vi "Read waveform file.vi"(7 "File IO parameters":T1={"Output Folder"=path "C:/Users/Abigail/Documents/Imperial Optical software/Optical Software Code Simplified/Output", "Error file"=path "Error Log.txt", "Config file"=path "Config.ini", "File prefix"="", "Waveform read"={"t0"=timestamp(0 s since 1904-01-01), "dt"=1.0, "Y"=[]}}, 8 "error in":errorcluster, 11 "Dataset name":string="DAQ (raw data)") -> (0 "error out":errorcluster, 2 "all rows":dbl[][](array[numeric]), 3 "Waveform":waveform(dbl))   [LabVIEW 2017, in "File IO.lvlib"]
uses:
  File IO.lvlib
  Controls/Params.ctl
  <vilib>/Utility/file.llb/Read Delimited Spreadsheet (DBL).vi
  <vilib>/Utility/file.llb/Read Delimited Spreadsheet (string).vi
panel:
  out "date last modified":timestamp
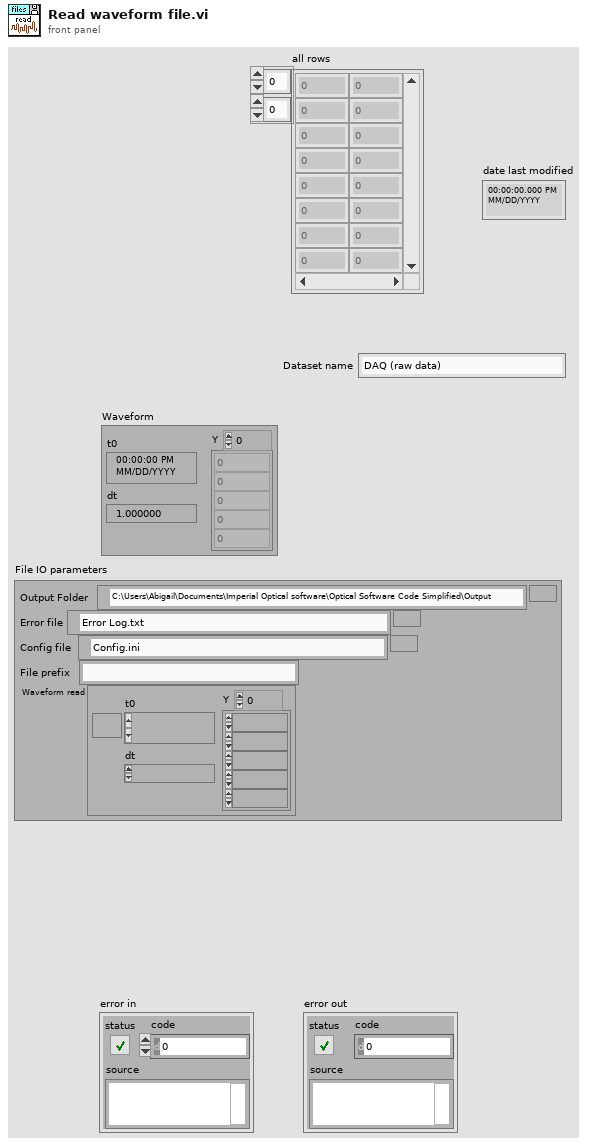
[diagram p1: front panel]
types:
  T1 = typedef "File IO.lvlib/Params.ctl" = cluster{"Output Folder":path, "Error file":path, "Config file":path, "File prefix":string, "Waveform read":waveform(dbl)}
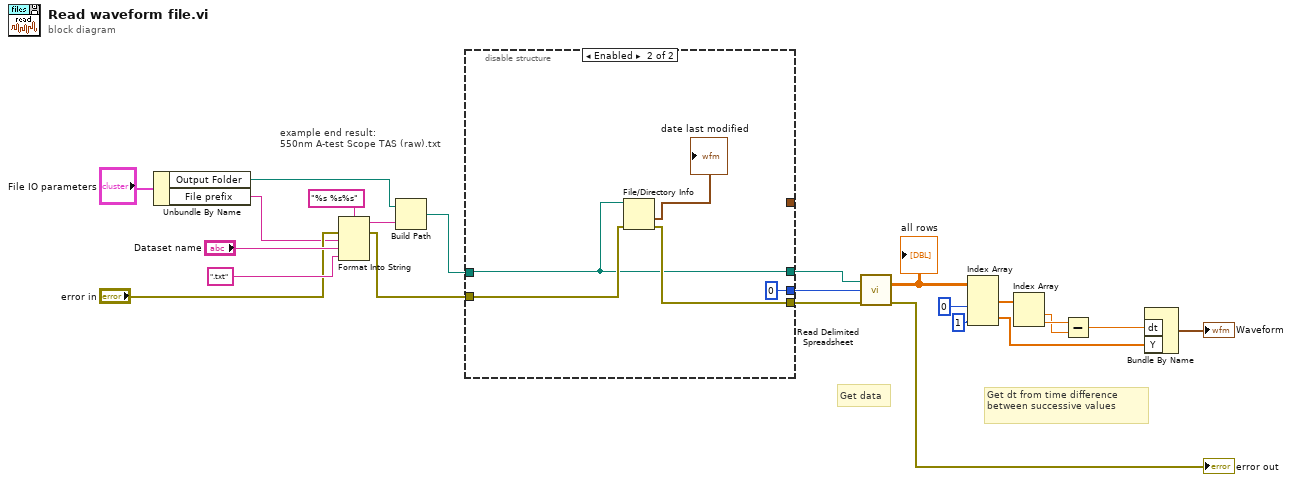
[diagram p0: block diagram]
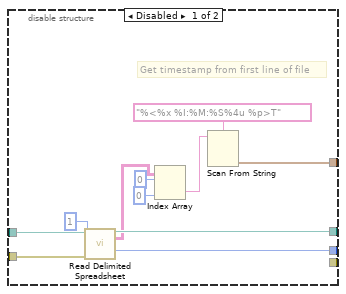
[diagram p2: hidden frame]
diagram:
  # "Get data"
  # "Get dt from time difference between successive values"
  # "example end result:\n550nm A-test Scope TAS (raw).txt"
  n1 = Unbundle By Name("File IO parameters") -> ("Output Folder"=w23:path, "File prefix"=w2:string)
  n2 = Format Into String(format string="%s %s%s", error in="error in", w2, "Dataset name", ".txt" ("Dataset name 2")) -> (resulting string=w19:string, error out=w16:errorcluster)  [unwired: 1 in]
  n3 = Build Path(base path=w23, name or relative path=w19) -> (appended path=w1:path)
  n4 = disable-structure shown="Enabled" {
    disable-tunnel: w1 -> [w34 w36]
    disable-tunnel: w16 -> [w33 w38]
    disable-tunnel: [w32 0 ("mark after read (chars.)")] -> w15
    disable-tunnel: [w31 w36] -> w14
    disable-tunnel: [w24 _] -> _
    disable-tunnel: [_ w37] -> w4
    frame Disabled {
      # "Get timestamp from first line of file"
      n5 = call-poly <vilib>:"Read Delimited Spreadsheet.vi"("file path (dialog if empty)"=w34, "number of rows (all:-1)"=1, "error in (no error)"=w33) -> ("new file path (Not A Path if cancelled)"=w31:path, "all rows"=w29:string[][], "mark after read (chars.)"=w32:i32)  [unwired: 7 in, 3 out]
      n6 = Index Array(array=w29, index (row)=0 ("disabled index (row)"), index (col)=0 ("disabled index (col)")) -> (element=w26:string)
      n7 = Scan From String(format string="%<%x %I:%M:%S%4u %p>T" ("time format string (%c)"), input string=w26) -> (output 1=w24:timestamp)  [unwired: 3 in, 3 out]
    }
    frame Enabled {
      n8 = File/Directory Info(path=w36, error in=w38) -> (last mod=→"date last modified":timestamp, error out=w37:errorcluster)  [unwired: 5 out]
    }
  }
  n9 = call-poly <vilib>:"Read Delimited Spreadsheet.vi"("file path (dialog if empty)"=w14, "start of read offset (chars.:0)"=w15, "error in (no error)"=w4) -> ("all rows"=w12:dbl[][], "error out"=→"error out":errorcluster)  [unwired: 7 in, 4 out]
  "all rows" <- w12
  n10 = Index Array(array=w12, index (col) #1=0 ("disabled index (col)"), index (col) #2=1 ("index (col)")) -> (element #1=w10:dbl[], element #2=w5:dbl[])  [unwired: 2 in]
  n11 = Index Array(array=w10) -> (element #1=w8:dbl, element #2=w9:dbl)  [unwired: 2 in]
  n12 = Subtract(x=w9, y=w8) -> (x-y=w7:dbl)
  n13 = Bundle By Name("dt"=w7, "Y"=w5) -> (→"Waveform":waveform(dbl))  [unwired: 1 in]
